vi "Shutdown.vi"(8 "Error In":errorcluster, 11 "Lexer In":refnum<class "Lexer.lvclass">) -> (0 "Error Out":errorcluster, 3 "Lexer Out":refnum<class "Lexer.lvclass">)   [LabVIEW 2018, in "Toolkit.lvlib" / "Lexer.lvclass"]
doc: "Safely destroys a Lexer object and cleans up any internally used resources. Once a Lexer object is destroyed, it cannot be used again and a new Lexer object must be created.\n\n<B>Lexer</B> - Represents an implementation capable of identifying tokens within a Mustache template."
uses:
  Lexer.lvclass
  Lexer.lvclass/Lexer.ctl
  Tokens/Token/Token.lvclass
  Support/Tag Types.ctl
  Support/States.ctl
  Type Definitions/Delimiters.ctl
  Toolkit.lvlib
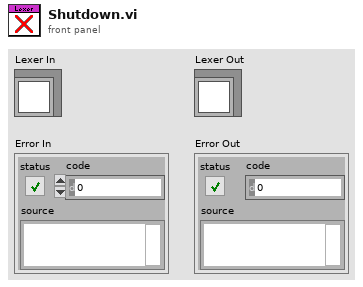
[diagram p1: front panel]
types:
  T1 = typedef "Toolkit.lvlib/Delimiters.ctl" = cluster{"Close":string, "Open":string}
  T2 = typedef "Toolkit.lvlib/Lexer.lvclass/States.ctl" = enum16{"Text", "Open Delimiter", "Tag Type", "Tag Key", "Close Delimiter"}
  T3 = typedef "Toolkit.lvlib/Lexer.lvclass/Tag Types.ctl" = enum16{"Escaped Variable", "{} Unescaped Variable", "& Unescaped Variable", "Begin Section", "Inverted Section", "End Section", "Comment", "Partial", "Set Delimiter"}
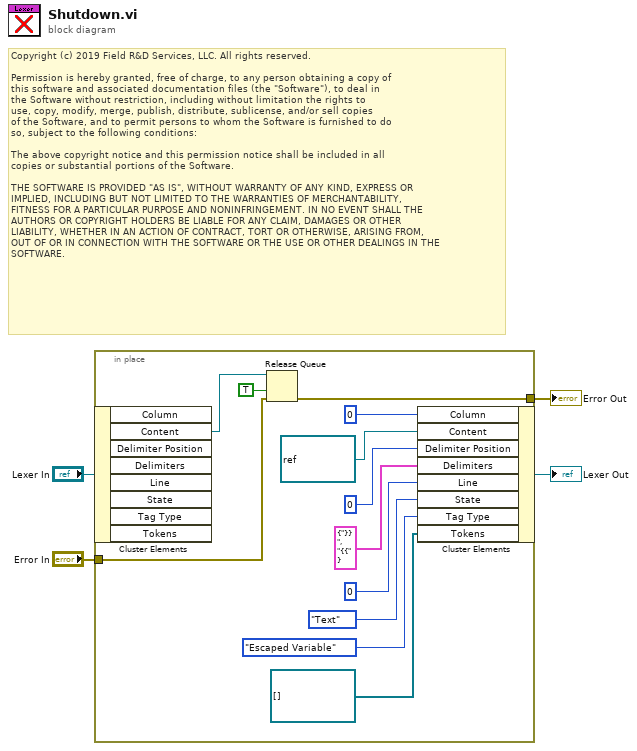
[diagram p0: block diagram]
diagram:
  # "Copyright (c) 2019 Field R&D Services, LLC. All rights reserved.\n\nPermission is hereby granted, free of charge, to any person obtaining a copy of\nthis software and associated documentation files (the \"Software\"), to deal in\nthe Software without restriction, including without limitation the rights to\nuse, copy, modify, merge, publish, distribute, sublicense, and/or sell copies\nof the Software, and to permit persons to whom the Software is furnished to do\nso, subject to the following conditions:\n\nThe above copyright notice and this permission notice shall be included in all\ncopies or substantial portions of the Software.\n\nTHE SOFTWARE IS PROVIDED \"AS IS\", WITHOUT WARRANTY OF ANY KIND, EXPRESS OR\nIMPLIED, INCLUDING BUT NOT LIMITED TO THE WARRANTIES OF MERCHANTABILITY,\nFITNESS FOR A PARTICULAR PURPOSE AND NONINFRINGEMENT. IN NO EVENT SHALL THE\nAUTHORS OR COPYRIGHT HOLDERS BE LIABLE FOR ANY CLAIM, DAMAGES OR OTHER\nLIABILITY, WHETHER IN AN ACTION OF CONTRACT, TORT OR OTHERWISE, ARISING FROM,\nOUT OF OR IN CONNECTION WITH THE SOFTWARE OR THE USE OR OTHER DEALINGS IN THE\nSOFTWARE."
  n1 = in-place {
    in-place-border: "Error In" -> [w16]
    in-place-border: [w15] -> w3
    n2 = in-place-cluster #1("Lexer In") -> ("Content"=w13:refnum<queue>)  [unwired: 7 out]
    n3 = Release Queue(queue=w13, force destroy? (F)=TRUE, error in (no error)=w16) -> (error out=w15:errorcluster)  [unwired: 2 out]
    n4 = in-place-cluster #1("Column"=u64 0, "Content"=refnum<queue> refnum, "Delimiter Position"=0, "Delimiters"=T1 {"Close"="}}", "Open"="{{"}, "Line"=u64 0, "State"=States."Text", "Tag Type"=Tag_Types."Escaped Variable", "Tokens"=refnum<class "Token.lvclass">[] []) -> (→"Lexer Out":refnum<class "Lexer.lvclass">)
  }
  "Error Out" <- w3
